vi "FTW-Test-JSON-ObjectKeys.vi"() -> (0 "Test Result":errorcluster)   [LabVIEW 2015]
uses:
  src/error/FTW-ERR-ThrowInfo.vi
  src/error/FTW-ERR-ThrowError.vi
  src/error/FTW-ERR-CallChain.vi
  src/string/FTW-STR-ReplaceWhitespace.vi
  src/string/FTW-STR-Array-Delimit.vi
panel:
  out "JSON String (UTF-8)":string
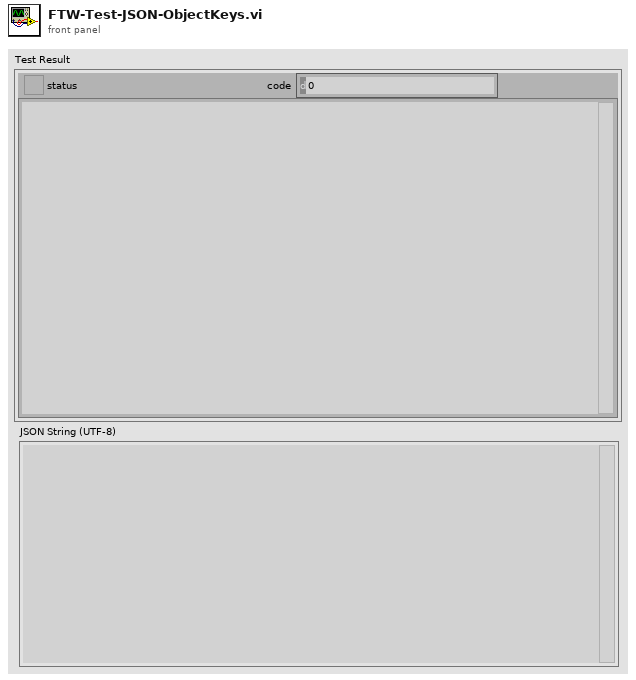
[diagram p1: front panel]
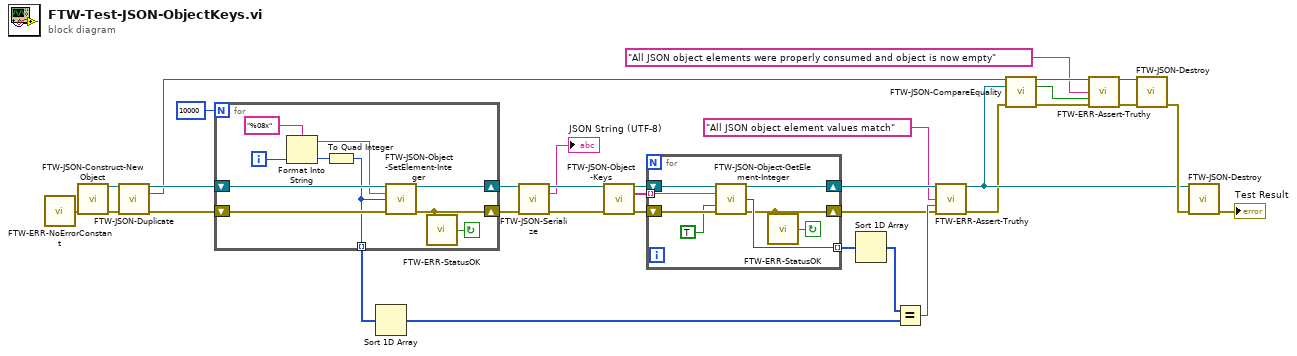
[diagram p0: block diagram]
diagram:
  n1 = call "FTW-ERR-NoErrorConstant.vi"() -> ("no error"=w31:errorcluster)
  n2 = call "FTW-JSON-Construct-NewObject.vi"("error in"=w31) -> ("JSON Object"=w27:refnum<data-value>, "error out"=w25:errorcluster)  [unwired: 13 in]
  n3 = call "FTW-JSON-Duplicate.vi"("JSON Object"=w27, "error in"=w25) -> ("JSON Object out"=w26:refnum<data-value>, "Duplicated JSON Object"=w22:refnum<data-value>, "error out"=w24:errorcluster)  [unwired: 11 in]
  n4 = for {
    N: 10000 -> [_]
    shift-right: [w33] -> w18
    shift-left: w24 -> [w38]
    shift-right: [w39] -> w20
    shift-left: w26 -> [w40]
    tunnel: [w34] -> w13 mode=indexing
    i -> [w37]
    stop <- w32 continue-if-true
    n5 = Format Into String(format string="%08x", w37) -> (resulting string=w36:string)  [unwired: 2 in, 1 out]
    n6 = To Quad Integer(1:w37) -> (0:w34:i64)
    n7 = call "FTW-JSON-Object-SetElement-Integer.vi"("JSON Object"=w40, "Key"=w36, "Value"=w34, "error in"=w38) -> ("JSON Object out"=w39:refnum<data-value>, "error out"=w33:errorcluster)  [unwired: 10 in]
    n8 = call "FTW-ERR-StatusOK.vi"("error to check"=w33) -> ("Status OK?"=w32:bool)
  }
  n9 = Sort 1D Array(array=w13) -> (sorted array=w12:i64[])
  n10 = call "FTW-JSON-Serialize.vi"("JSON Object"=w20, "error in"=w18) -> ("JSON Object out"=w19:refnum<data-value>, "JSON String (UTF-8)"=→"JSON String (UTF-8)":string, "error out"=w17:errorcluster)  [unwired: 11 in]
  n11 = call "FTW-JSON-Object-Keys.vi"("JSON Object"=w19, "error in"=w17) -> ("JSON Object out"=w30:refnum<data-value>, "Keys"=w29:string[], "error out"=w28:errorcluster)  [unwired: 11 in]
  n12 = for {
    tunnel: w29 -> [w46] mode=indexing
    shift-right: [w42] -> w8
    shift-left: w28 -> [w47]
    tunnel: [w45] -> w15 mode=indexing
    shift-right: [w44] -> w10
    shift-left: w30 -> [w48]
    stop <- w43 continue-if-true
    n13 = call "FTW-JSON-Object-GetElement-Integer.vi"("JSON Object"=w48, "Key"=w46, "Consume Value"=TRUE, "error in"=w47) -> ("JSON Object out"=w44:refnum<data-value>, "Value"=w45:i64, "error out"=w42:errorcluster)  [unwired: 8 in, 1 out]
    n14 = call "FTW-ERR-StatusOK.vi"("error to check"=w42) -> ("Status OK?"=w43:bool)
  }
  n15 = Sort 1D Array(array=w15) -> (sorted array=w14:i64[])
  n16 = Equal?(x=w14, y=w12) -> (x = y?=w9:bool)
  n17 = call "FTW-ERR-Assert-Truthy.vi"("Assertion"="All JSON object element values match", "Assertion holds true?"=w9, "error in"=w8) -> ("error out"=w7:errorcluster)  [unwired: 12 in]
  n18 = call "FTW-JSON-CompareEquality.vi"("JSON Object"=w22, "JSON Object to Compare"=w10, "error in"=w7) -> ("JSON Object out"=w11:refnum<data-value>, "Equal?"=w3:bool, "error out"=w5:errorcluster)  [unwired: 10 in]
  n19 = call "FTW-ERR-Assert-Truthy.vi"("Assertion"="All JSON object elements were properly consumed and object is now empty", "Assertion holds true?"=w3, "error in"=w5) -> ("error out"=w4:errorcluster)  [unwired: 12 in]
  n20 = call "FTW-JSON-Destroy.vi"("JSON Object"=w11, "error in"=w4) -> ("error out"=w21:errorcluster)  [unwired: 13 in]
  n21 = call "FTW-JSON-Destroy.vi"("JSON Object"=w10, "error in"=w21) -> ("error out"=→"Test Result":errorcluster)  [unwired: 13 in]
